vi "PCO_SetPowerDownMode.vi"(8 "error in (no error)":errorcluster {"code" format="%x"}, 10 "wPowerDownMode":u16(ring) items=["auto", "user"], 11 "ph":u64) -> (0 "error out":errorcluster {"code" format="%x"}, 2 "ErrorMessage":i32 format="%x", 3 "ph out":u64)   [LabVIEW 2020, in "SDK.lvlib" / "TimingControl.lvlib"]
doc: "<b>Description:</b>\nThis function does set the power down mode of the camera. Descriptor flag wPowerDownModeDESC determines, if power down mode is available and if the camera can switch the sensor into power down mode for reduced dark current during long exposure times. By default power down mode [auto] is selected and the camera does select the threshhold time best suitable for the installed sensor. When power down mode is set to [user] the threshhold time can be set through function PCO_SetUserPowerDownTime.\n\n<b>Supported camera type:</b>\npco.1600, pco.2000, pco.4000\n\n<b>Descriptor dependency:</b>\nwPowerDownModeDESC"
uses:
  TimingControl.lvlib
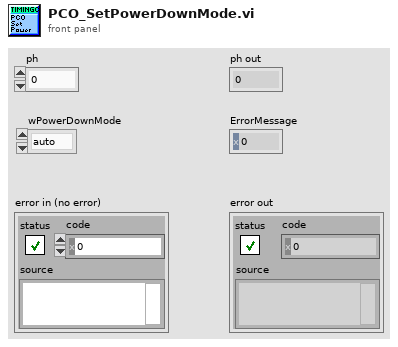
[diagram p1: front panel]
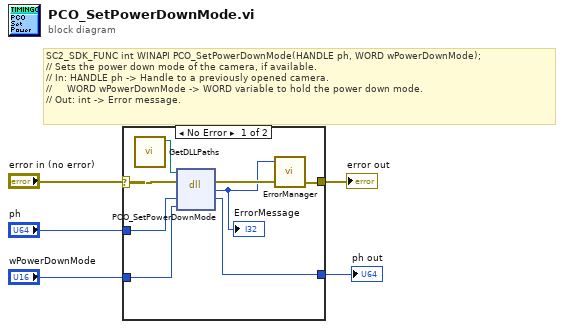
[diagram p0: block diagram]
diagram:
  # "SC2_SDK_FUNC int WINAPI PCO_SetPowerDownMode(HANDLE ph, WORD wPowerDownMode);\n// Sets the power down mode of the camera, if available.\n// In: HANDLE ph -> Handle to a previously opened camera.\n//     WORD wPowerDownMode -> WORD variable to hold the power down mode.\n// Out: int -> Error message."
  n1 = case shown="No Error" "error in (no error)" {
    selector: "error in (no error)" -> [w10 w15]
    tunnel: "ph" -> [w13 w14]
    tunnel: [w12 w14] -> w4
    tunnel: "wPowerDownMode" -> [w11 _]
    tunnel: [w8 w15] -> w2
    frame No Error {
      n2 = call "GetDLLPaths.vi"() -> ("SC2_Cam_Path"=w6:path)  [unwired: 9 in, 2 out]
      n3 = dll-call lib="?" fn="PCO_SetPowerDownMode"(path in=w6, error in=w10, "ph"=w13, "wPowerDownMode"=w11) -> (error out=w9:errorcluster, "return type"=w7:i32, "ph"=w12:u64)  [unwired: 2 in, 1 out]
      "ErrorMessage" <- w7
      n4 = call "ErrorManager.vi"("error in (no error)"=w9, "error code"=w7) -> ("error out"=w8:errorcluster)  [unwired: 3 in]
    }
    frame Error {
    }
  }
  "ph out" <- w4
  "error out" <- w2
